vi "Database-Init.vi"(8 "error in":errorcluster, 11 "Idx":i32) -> (0 "error out":errorcluster)   [LabVIEW 2016]
uses:
  Database.Action.ctl
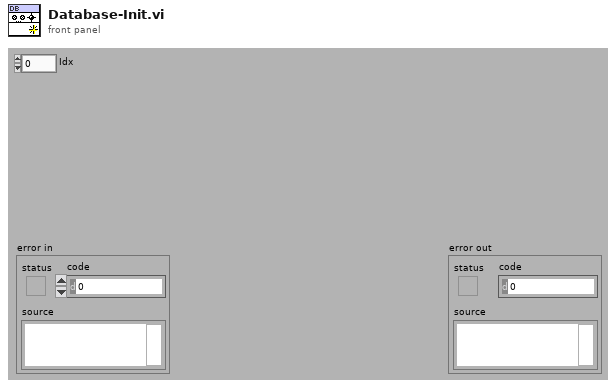
[diagram p1: front panel]
types:
  T1 = typedef "Database.Action.ctl" = enum32{"idle", "constructor", "destructor", "--- DB ---", "Setup", "Init", "ExportData", "Changeover", "GetPrevStatus", "GetThisStatus", "GetComponent"}
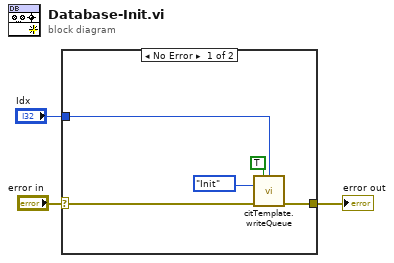
[diagram p0: block diagram]
diagram:
  n1 = case shown="No Error" "error in" {
    selector: "error in" -> [w7 w9]
    tunnel: [w8 w9] -> w2
    tunnel: "Idx" -> [w4 _]
    frame No Error {
      n2 = call "citTemplate.writeQueue.vi"("High priority (F)"=TRUE, "instance (0)"=w4, "event in (if not connected:all statemachine with data event)"=Database.Action."Init" ("Action"), "error in (no error)"=w7) -> ("error out"=w8:errorcluster)  [unwired: 11 in]
    }
    frame Error {
    }
  }
  "error out" <- w2
